vi "InitCam3010.vi"(7 "error in (no error)":errorcluster) -> (0 "error out":errorcluster)   [LabVIEW 2015, in "ESLSCDLL.lvlib"]
uses:
  ESLSCDLL.lvlib
  Globals.vi
  ESLSCDLL.dll
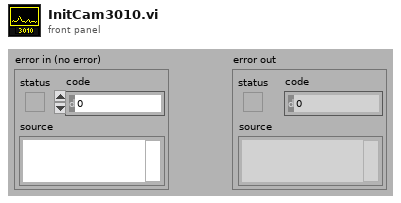
[diagram p1: front panel]
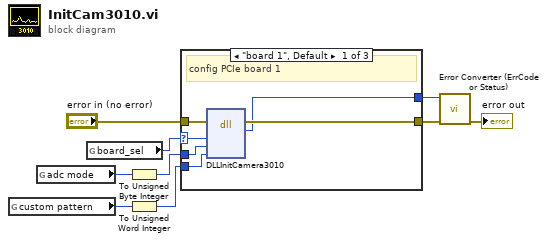
[diagram p0: block diagram]
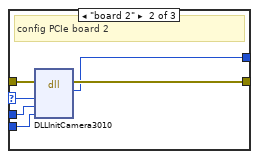
[diagram p2: hidden frame]
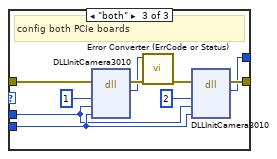
[diagram p3: hidden frame]
diagram:
  n1 = global read "Globals.vi" "custom pattern"() -> (w3:u32)
  n2 = global read "Globals.vi" "adc mode"() -> (w4:enum16{"normal", "ramp", "custom pattern"})
  n3 = global read "Globals.vi" "board_sel"() -> (w5:enum32{"0", "board 1", "board 2", "both"})
  n4 = To Unsigned Byte Integer(number=w4) -> (unsigned 8bit integer=w2:u8)
  n5 = To Unsigned Word Integer(number=w3) -> (unsigned 16bit integer=w1:u16)
  n6 = case shown="\"board 1\", Default" w5 {
    selector: w5 -> [w15 w21 _]
    tunnel: w2 -> [w14 w19 w30]
    tunnel: w1 -> [w13 w20 w31]
    tunnel: "error in (no error)" -> [w12 w18 w27]
    tunnel: [w11 w17 w23] -> w8
    tunnel: [w10 w16 w22] -> w7
    frame "board 1", Default {
      # "config PCIe board 1"
      n7 = dll-call lib="C:/ENTW/PCIE/LV64/board.vis/ESLSCDLL.dll" fn="DLLInitCamera3010" ("lwlscdll.dll:DLLWriteLongS0")(error in=w12, "drvno"=w15, "adc_mode"=w14, "custom_pattern"=w13) -> (error out=w11:errorcluster, "es_status_codes"=w10:i32)  [unwired: 5 in, 1 out]
    }
    frame "board 2" {
      # "config PCIe board 2"
      n8 = dll-call lib="C:/ENTW/PCIE/LV64/board.vis/ESLSCDLL.dll" fn="DLLInitCamera3010" ("lwlscdll.dll:DLLWriteLongS0")(error in=w18, "drvno"=w21, "adc_mode"=w19, "custom_pattern"=w20) -> (error out=w17:errorcluster, "es_status_codes"=w16:i32)  [unwired: 5 in, 1 out]
    }
    frame "both" {
      # "config both PCIe boards"
      n9 = dll-call lib="C:/ENTW/PCIE/LV64/board.vis/ESLSCDLL.dll" fn="DLLInitCamera3010" ("lwlscdll.dll:DLLWriteLongS0")(error in=w27, "drvno"=u32 1, "adc_mode"=w30, "custom_pattern"=w31) -> (error out=w26:errorcluster, "es_status_codes"=w25:i32)  [unwired: 5 in, 1 out]
      n10 = call "Error Converter (ErrCode or Status).vi"("error in (no error)"=w26, "error code"=w25) -> ("error out"=w24:errorcluster)  [unwired: 9 in]
      n11 = dll-call lib="C:/ENTW/PCIE/LV64/board.vis/ESLSCDLL.dll" fn="DLLInitCamera3010" ("lwlscdll.dll:DLLWriteLongS0")(error in=w24, "drvno"=u32 2, "adc_mode"=w30, "custom_pattern"=w31) -> (error out=w23:errorcluster, "es_status_codes"=w22:i32)  [unwired: 5 in, 1 out]
    }
  }
  n12 = call "Error Converter (ErrCode or Status).vi"("error in (no error)"=w8, "error code"=w7) -> ("error out"=→"error out":errorcluster)  [unwired: 9 in]
